vi "HGF_SVService.appendData2Variant.vi"(0 "initData":variant, 1 "typeDescriptor":string, 2 "defaultData":variant, 3 "defaultQuality":i32, 4 "variable":string, 5 "error in (no error)":errorcluster, 7 "protocol":enum8{"psp", "opc"}(ring)) -> (14 "dup initData":variant, 19 "error out":errorcluster)   [LabVIEW 2012, in "HGF_SV.lvlib" / "HGF_SVService.lvclass"]
uses:
  HGF_SVService.lvclass
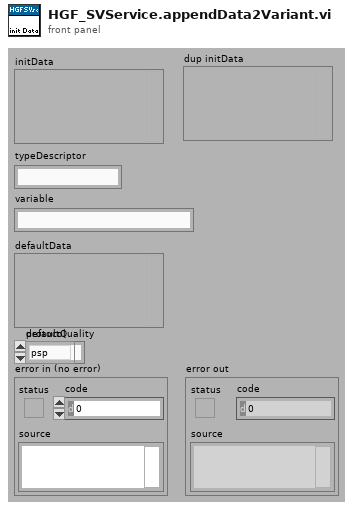
[diagram p1: front panel]
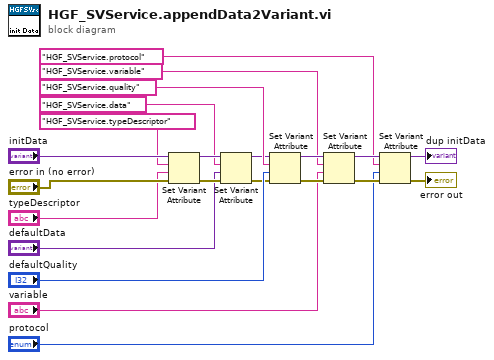
[diagram p0: block diagram]
diagram:
  n1 = Set Variant Attribute(Variant="initData", name="HGF_SVService.typeDescriptor", value="typeDescriptor", error in="error in (no error)") -> (Variant out=w17:variant, error out=w18:errorcluster)  [unwired: 1 out]
  n2 = Set Variant Attribute(Variant=w17, name="HGF_SVService.data", value="defaultData", error in=w18) -> (Variant out=w14:variant, error out=w13:errorcluster)  [unwired: 1 out]
  n3 = Set Variant Attribute(Variant=w14, name="HGF_SVService.quality", value="defaultQuality", error in=w13) -> (Variant out=w11:variant, error out=w10:errorcluster)  [unwired: 1 out]
  n4 = Set Variant Attribute(Variant=w11, name="HGF_SVService.variable", value="variable", error in=w10) -> (Variant out=w7:variant, error out=w6:errorcluster)  [unwired: 1 out]
  n5 = Set Variant Attribute(Variant=w7, name="HGF_SVService.protocol", value="protocol", error in=w6) -> (Variant out=→"dup initData":variant, error out=→"error out":errorcluster)  [unwired: 1 out]
